vi "Result_Test.vi"(8 "error in (no error)":errorcluster caption="entrée d'erreur (pas d'erreur)", 11 "Nodon_Get_BP_Status IN":refnum<class "Nodon_Get_BP_Status.lvclass">) -> (0 "error out":errorcluster caption="sortie d'erreur", 3 "Nodon_Get_BP_Status OUT":refnum<class "Nodon_Get_BP_Status.lvclass">)   [LabVIEW 2020, in "Library Test.lvlib" / "Nodon_Get_BP_Status.lvclass"]
uses:
  Nodon_Get_BP_Status.lvclass
  C:/Users/ngarcin/OneDrive - Altyor/Standard TB/Class/Test/Test (Default)/Test (Default).lvclass
  JSON API/JSON Value/Set from JSON string.vi
  JSON API/JSON Value/JSON Value.lvclass
  Nodon_Send_Command_UART.lvclass
  Nodon_Get_BP_Status.lvclass/Nodon_Get_BP_Status.ctl
  JSON API/Variant JSON/Variant JSON.lvlib
  JSON API/Get Polymorphic/JSON GetSet.lvlib
  Commun VI/Library Commun.lvlib
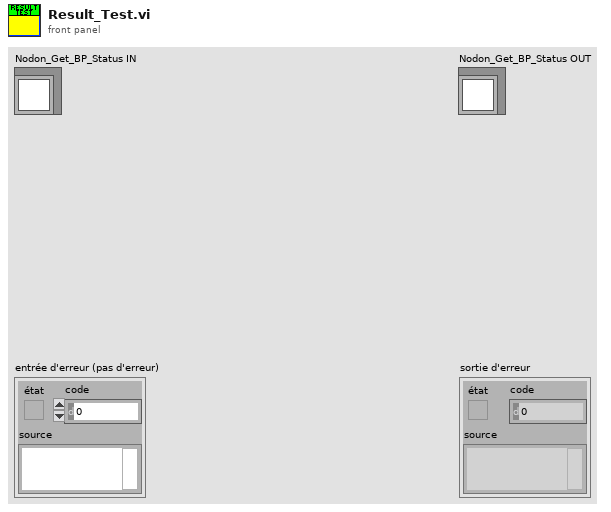
[diagram p1: front panel]
types:
  T1 = cluster{"Commande Type":string, "Command ID":string, "Data":string, "Error":string}
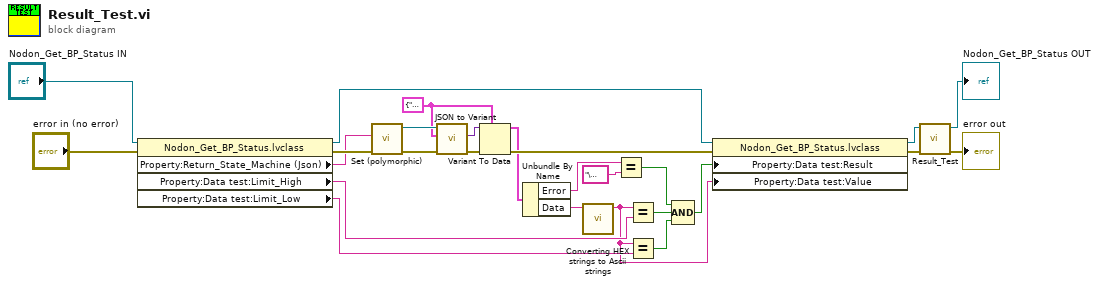
[diagram p0: block diagram]
diagram:
  w13 = T1 {"Commande Type"="", "Command ID"="", "Data"="", "Error"=""}
  n1 = property class="Nodon_Get_BP_Status.lvclass"(reference="Nodon_Get_BP_Status IN", error in="error in (no error)") -> (reference out=w24:refnum<class "Nodon_Get_BP_Status.lvclass">, error out=w19:errorcluster, "Property:Return_State_Machine (Json)"=w17:string, "Property:Data test:Limit_High"=w6:string, "Property:Data test:Limit_Low"=w5:string)
  n2 = call-poly "Set (polymorphic).vi"("error in (no error)"=w19, "JSON stream"=w17) -> ("error out"=w21:errorcluster, "JSON Value out"=w23:refnum<class "JSON Value.lvclass">)  [unwired: 7 in, 1 out]
  n3 = call "JSON to Variant.vi"("error in (no error)"=w21, "Variant (Data Type)"=w13, "JSON Value"=w23) -> ("error out"=w22:errorcluster, "Variant out"=w20:variant)  [unwired: 7 in]
  n4 = Variant To Data(error in=w22, type=w13, Variant=w20) -> (data=w16:T1, error out=w18:errorcluster)
  n5 = Unbundle By Name(w16) -> ("Error"=w15:string, "Data"=w8:string)
  n6 = call "Converting HEX strings to Ascii strings.vi"("chaîne IN"=w8) -> ("Chaîne OUT"=w4:string)  [unwired: 9 in, 1 out]
  n7 = Equal?(x=w15, y="\u0000") -> (x = y?=w2:bool)
  n8 = Equal?(x=w4, y=w6) -> (x = y?=w7:bool)
  n9 = Equal?(x=w4, y=w5) -> (x = y?=w3:bool)
  n10 = Compound Arithmetic op=AND ("Opérateur arithmétique")(w2, w7, w3) -> (w1:bool)
  n11 = property class="Nodon_Get_BP_Status.lvclass"(reference=w24, error in=w18, "Property:Data test:Result"=w1, "Property:Data test:Value"=w4) -> (reference out=w10:refnum<class "Nodon_Get_BP_Status.lvclass">, error out=w9:errorcluster)
  n12 = call-parent "Result_Test.vi"("error in (no error)"=w9, "Get_Voltage en entrée"=w10) -> ("error out"=→"error out":errorcluster, "Get_Voltage en sortie"=→"Nodon_Get_BP_Status OUT":refnum<class "Nodon_Get_BP_Status.lvclass">)  [unwired: 8 in]
